vi "Motor Control SubVI.vi"(9 "Speed M2":dbl(slide) scale=-1.0..1.0, 10 "Speed M1":dbl(slide) scale=-1.0..1.0, 11 "Speed M0":dbl(slide) scale=-1.0..1.0) -> (2 "Motor Error":errorcluster)   [LabVIEW 2018]
uses:
  <vilib>/Studica/Studica Toolkit/Background/Mxp Selection.ctl
panel:
  in  "stop":bool
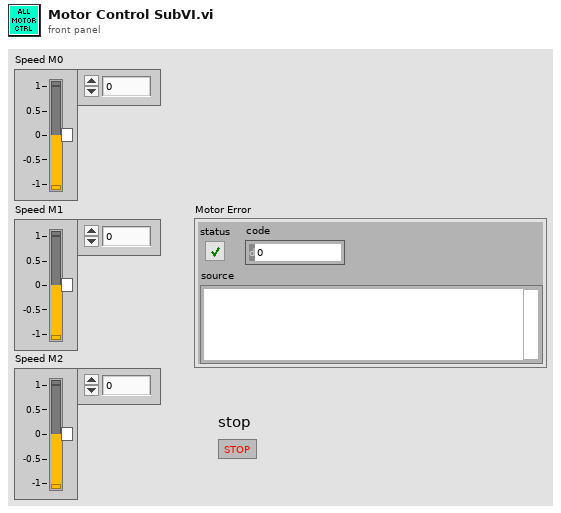
[diagram p1: front panel]
types:
  T1 = typedef "Mxp Selection.ctl" = enum16{"MXP A", "MXP B"}
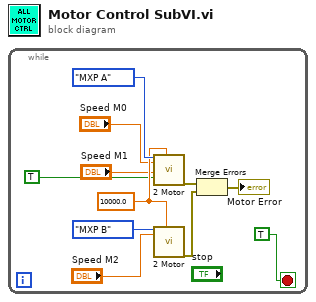
[diagram p0: block diagram]
diagram:
  n1 = while {
    stop <- TRUE stop-if-true
    w9 = 10000.0 ("Frequency [Hz]")
    n2 = call <vilib>:"2 Motor.vi"("Mxp Side"=Mxp_Selection."MXP A", "Speed M0"="Speed M0", "Speed M1"="Speed M1", "Invert M1"=TRUE, "Frequency [Hz]"=w9) -> ("error out"=w5:errorcluster)  [unwired: 14 in]
    n3 = call <vilib>:"2 Motor.vi"("Mxp Side"=Mxp_Selection."MXP B", "Speed M0"="Speed M2", "Frequency [Hz]"=w9) -> ("error out"=w4:errorcluster)  [unwired: 16 in]
    n4 = Merge Errors(w5, w4) -> (→"Motor Error":errorcluster)
  }
